vi "Paramater_set.vi"(6 "ON/OFF":bool, 8 "error in (no error)":errorcluster, 9 "Current":i32, 10 "Voltage":i32, 11 "IT6932A in":refnum<class "IT6932A.lvclass">) -> (0 "error out":errorcluster, 3 "IT6932A out":refnum<class "IT6932A.lvclass">)   [LabVIEW 2023, in "IT6932A.lvclass"]
uses:
  IT6932A.lvclass
  IT6932A.lvclass/IT6932A.ctl
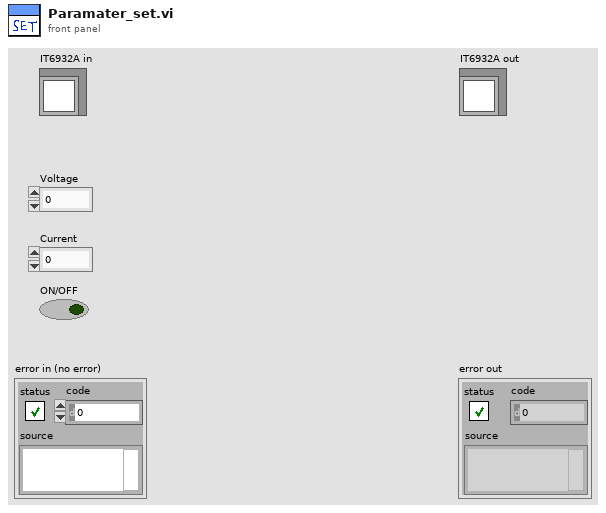
[diagram p1: front panel]
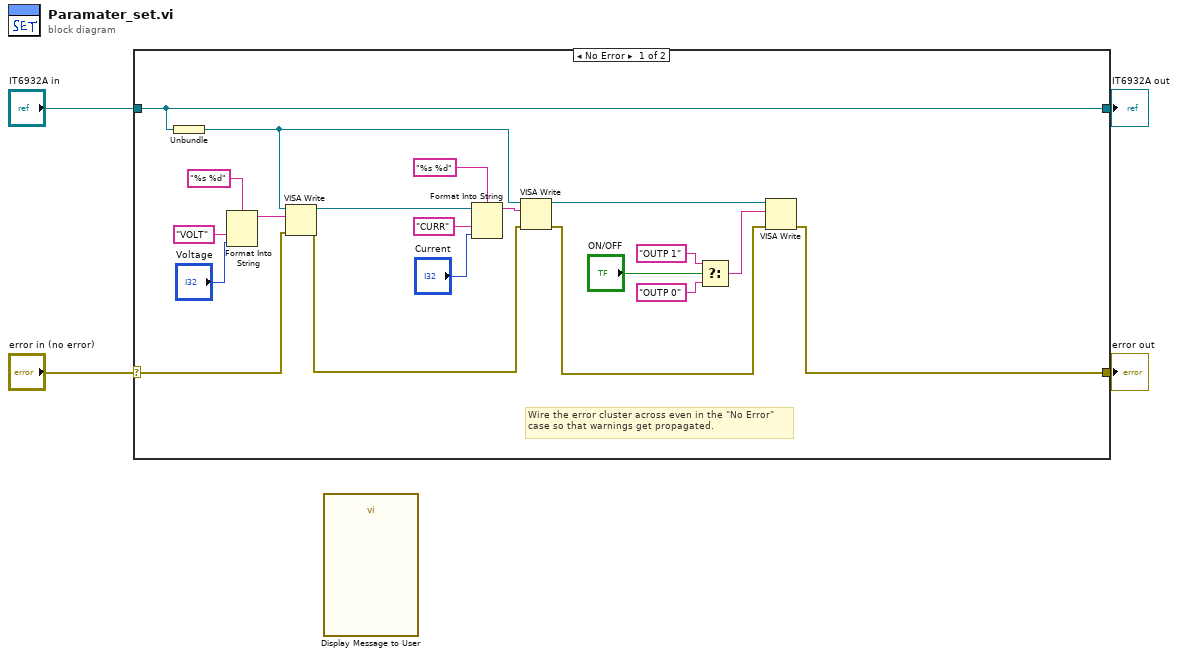
[diagram p0: block diagram]
diagram:
  n1 = case shown="No Error" "error in (no error)" {
    selector: "error in (no error)" -> [w16 w26]
    tunnel: [w6 w26] -> w3
    tunnel: [w17 w25] -> w1
    tunnel: "IT6932A in" -> [w17 w25]
    frame No Error {
      # "Wire the error cluster across even in the \"No Error\"\ncase so that warnings get propagated."
      n2 = Unbundle(w17) -> (w14:refnum<visa-resource-name>)
      n3 = Format Into String(format string="%s %d", "VOLT" ("write buffer"), "Voltage") -> (resulting string=w22:string)  [unwired: 2 in, 1 out]
      n4 = VISA Write(VISA resource name=w14, write buffer=w22, error in (no error)=w16) -> (VISA resource name out=w15:refnum<visa-resource-name>, error out=w12:errorcluster)  [unwired: 1 out]
      n5 = Format Into String(format string="%s %d", initial string=w15, "CURR" ("write buffer"), "Current") -> (resulting string=w13:string)  [unwired: 1 in, 1 out]
      n6 = VISA Write(VISA resource name=w14, write buffer=w13, error in (no error)=w12) -> (VISA resource name out=w11:refnum<visa-resource-name>, error out=w7:errorcluster)  [unwired: 1 out]
      n7 = Select(t="OUTP 1" ("write buffer"), s="ON/OFF", f="OUTP 0" ("write buffer")) -> (s? t:f=w8:string)
      n8 = VISA Write(VISA resource name=w11, write buffer=w8, error in (no error)=w7) -> (error out=w6:errorcluster)  [unwired: 2 out]
    }
    frame Error {
    }
  }
  "error out" <- w3
  "IT6932A out" <- w1
  n9 = call "Display Message to User"() -> ()  [unwired: 10 in, 2 out]
